vi "updateState.vi"(8 "error in (no error)":errorcluster, 9 "calibratedValues":dbl[](array[numeric]), 10 "channel_addresses":string[](array[string]), 11 "DigitalOutput in":refnum<class "DigitalOutput.lvclass">) -> (0 "error out":errorcluster, 3 "DigitalOutput out":refnum<class "DigitalOutput.lvclass">)   [LabVIEW 2009, in "Hardware.lvlib" / "Channels.lvlib" / "DigitalOutput.lvclass"]
uses:
  DigitalOutput.lvclass
  DigitalOutput.lvclass/DigitalOutput.ctl
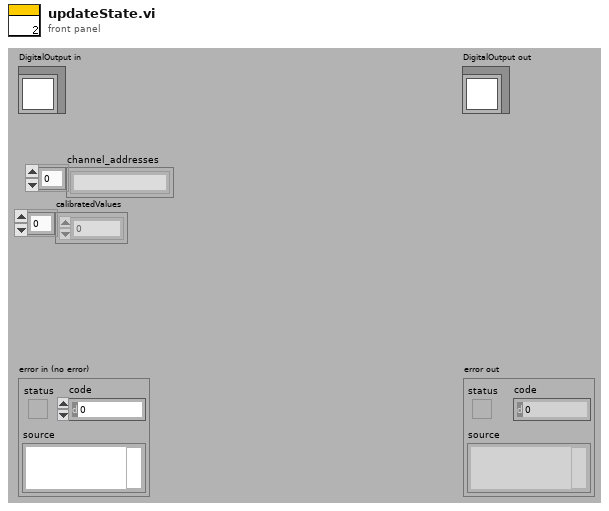
[diagram p1: front panel]
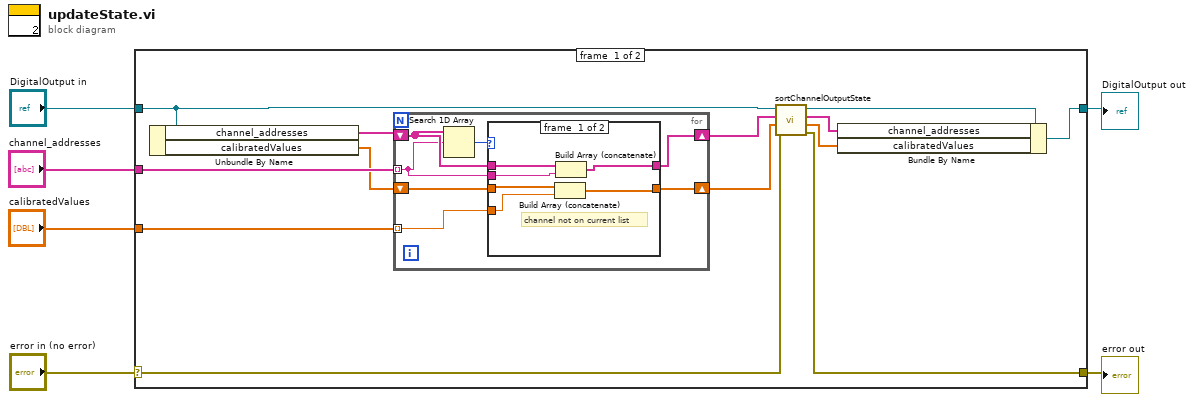
[diagram p0: block diagram]
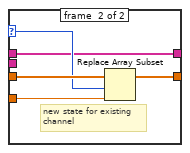
[diagram p2: hidden frame]
diagram:
  n1 = case shown="No Error" "error in (no error)" {
    selector: "error in (no error)" -> [w12 w39]
    tunnel: [w11 w39] -> w5
    tunnel: [w7 w38] -> w3
    tunnel: "DigitalOutput in" -> [w15 w38]
    tunnel: "channel_addresses" -> [w19 _]
    tunnel: "calibratedValues" -> [w17 _]
    frame #0 {
      n2 = Unbundle By Name(w15) -> ("channel_addresses"=w18:string[], "calibratedValues"=w16:dbl[])
      n3 = for {
        tunnel: w19 -> [w21] mode=indexing
        tunnel: w17 -> [w24] mode=indexing
        shift-right: [w23] -> w13
        shift-left: w16 -> [w25]
        shift-right: [w20] -> w14
        shift-left: w18 -> [w22]
        n4 = Search 1D Array(1D array=w22, element=w21) -> (index of element=w26:i32)  [unwired: 1 in]
        n5 = case shown="Default" w26 {
          selector: w26 -> [_ w35]
          tunnel: w25 -> [w32 w37]
          tunnel: w24 -> [w31 w36]
          tunnel: [w30 w34] -> w23
          tunnel: w22 -> [w29 w33]
          tunnel: w21 -> [w28 _]
          tunnel: [w27 w33] -> w20
          frame #0 {
            # "channel not on current list"
            n6 = Build Array (concatenate)(w32, w31) -> (w30:dbl[])
            n7 = Build Array (concatenate)(w29, w28) -> (w27:string[])
          }
          frame #1 {
            # "new state for existing \nchannel"
            n8 = Replace Array Subset(array=w37, new element=w36, index=w35) -> (w34:dbl[])
          }
        }
      }
      n9 = call "sortChannelOutputState.vi"("error in (no error)"=w12, "calibratedValues"=w13, "channel_addresses"=w14, "DigitalOutput in"=w15) -> ("error out"=w11:errorcluster, "calibratedValues out"=w9:dbl[], "channel_addresses out"=w10:string[], "DigitalOutput out"=w8:refnum<class "DigitalOutput.lvclass">)  [unwired: 4 in]
      n10 = Bundle By Name(cluster=w8, "channel_addresses"=w10, "calibratedValues"=w9) -> (w7:refnum<class "DigitalOutput.lvclass">)
    }
    frame #1 {
    }
  }
  "error out" <- w5
  "DigitalOutput out" <- w3
